vi "Get SMO Public API.vi"(8 "error in (no error)":errorcluster, 11 "Instrument.Framework-Template in":refnum<class "Instrument.Framework-Template.lvclass">) -> (0 "error out":errorcluster, 2 "Commands":string[](array[string]), 3 "Instrument.Framework-Template out":refnum<class "Instrument.Framework-Template.lvclass">)   [LabVIEW 2019, in "Instrument.Framework-Template.lvclass"]
uses:
  Instrument.Framework-Template.lvclass
  Instrument Types/SCPI/Instrument.SCPI.lvclass
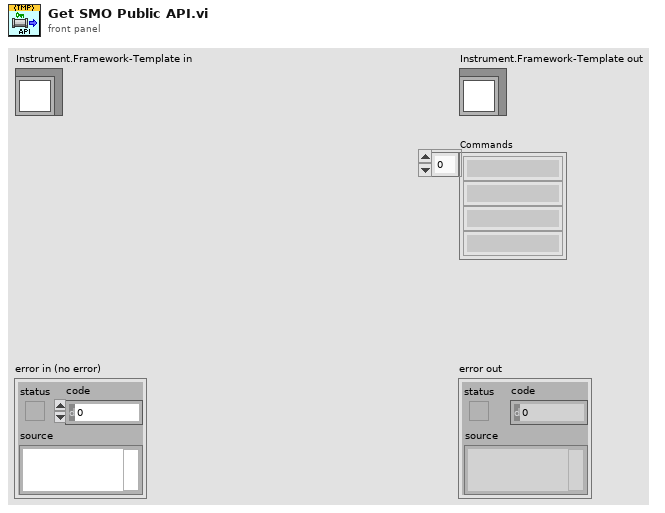
[diagram p1: front panel]
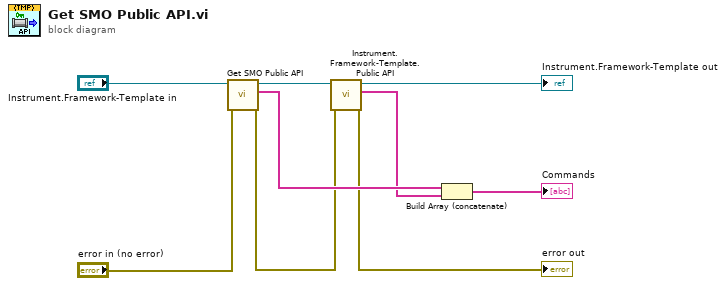
[diagram p0: block diagram]
diagram:
  n1 = call-parent "Get SMO Public API.vi"("error in (no error)"="error in (no error)", "Instrument in"="Instrument.Framework-Template in") -> ("error out"=w3:errorcluster, "commands"=w8:string[], "Instrument out"=w4:refnum<class "Instrument.Framework-Template.lvclass">)  [unwired: 7 in]
  n2 = call "Instrument.Framework-Template.Public API.vi"("error in (no error)"=w3, "Instrument.Framework-Template in"=w4) -> ("error out"=→"error out":errorcluster, "commands (this level)"=w5:string[], "Instrument.Framework-Template out"=→"Instrument.Framework-Template out":refnum<class "Instrument.Framework-Template.lvclass">)  [unwired: 7 in]
  n3 = Build Array (concatenate)(w8, w5) -> (→"Commands":string[])
